vi "write_TIFF_multipage.vi"(6 "description tag":string, 8 "error in (no error)":errorcluster, 10 "description file":path, 11 "path in":path) -> (0 "error out":errorcluster, 3 "path out":path)   [LabVIEW 2010, in "TIFFManagement.lvlib"]
uses:
  TIFFManagement.lvlib
  VisualCPP/Release/TIFFManagement.dll
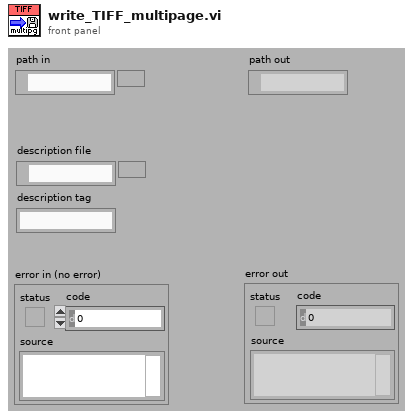
[diagram p1: front panel]
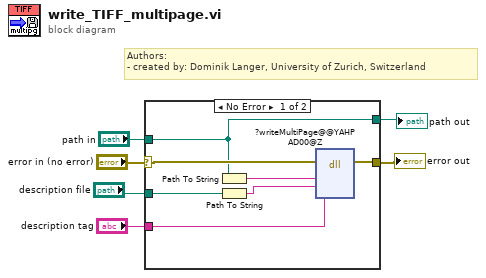
[diagram p0: block diagram]
diagram:
  # "Authors: \n- created by: Dominik Langer, University of Zurich, Switzerland"
  n1 = case shown="No Error" "error in (no error)" {
    selector: "error in (no error)" -> [w11 w15]
    tunnel: "path in" -> [w8 w14]
    tunnel: [w10 w15] -> w4
    tunnel: [w8 w14] -> w3
    tunnel: "description file" -> [w9 _]
    tunnel: "description tag" -> [w7 _]
    frame No Error {
      n2 = Path To String(path=w8) -> (string=w13:string)
      n3 = Path To String(path=w9) -> (string=w12:string)
      n4 = dll-call lib="C:/helioscan/common/libraries/TIFFManagement/VisualCPP/Release/TIFFManagement.dll" fn="?writeMultiPage@@YAHPAD00@Z"(error in=w11, "path"=w13, "description file path"=w12, "description"=w7) -> (error out=w10:errorcluster)  [unwired: 6 in, 1 out]
    }
    frame Error {
    }
  }
  "error out" <- w4
  "path out" <- w3
